vi "Set Priority.vi"(10 "Priority":i32=100, 11 "Thread Parameters in":refnum<class "Thread Parameters.lvclass">) -> (3 "Thread Parameters out":refnum<class "Thread Parameters.lvclass">)   [LabVIEW 2017, in "Data Sharing Framework Core.lvlib" / "Data Sharing Framework Engine.lvlib" / "Thread Parameters.lvclass"]
uses:
  Thread Parameters.lvclass
  Thread Parameters.lvclass/Thread Parameters.ctl
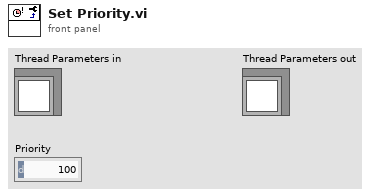
[diagram p1: front panel]
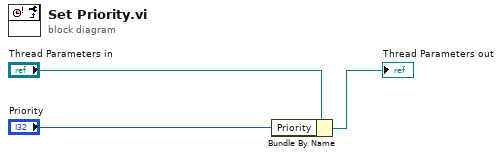
[diagram p0: block diagram]
diagram:
  n1 = Bundle By Name(cluster="Thread Parameters in", "Priority"="Priority") -> (→"Thread Parameters out":refnum<class "Thread Parameters.lvclass">)
